vi "Destroy.vi"(8 "Error In":errorcluster, 11 "reference in":refnum<class "VdAnalogInput_Simulated.lvclass">) -> (0 "Error Out":errorcluster, 3 "reference out":refnum<class "VdAnalogInput_Simulated.lvclass">)   [LabVIEW 2020, in "VdAnalogInput_Simulated.lvclass"]
uses:
  VdAnalogInput_Simulated.lvclass
  VdAnalogInput_class/VdAnalogInput.lvclass
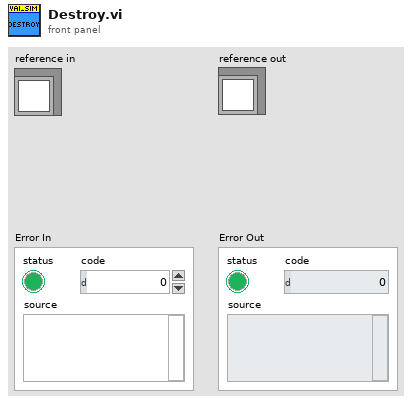
[diagram p1: front panel]
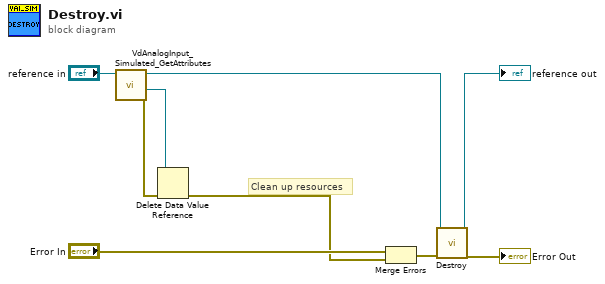
[diagram p0: block diagram]
diagram:
  # "Clean up resources"
  n1 = call "VdAnalogInput_Simulated_GetAttributes.vi"("reference in"="reference in") -> ("error out"=w7:errorcluster, "DataRef"=w5:refnum<data-value>, "reference out"=w6:refnum<class "VdAnalogInput_Simulated.lvclass">)  [unwired: 7 in, 1 out]
  n2 = Delete Data Value Reference(data value reference=w5, error in=w7) -> (error out=w1:errorcluster)  [unwired: 1 out]
  n3 = Merge Errors("Error In", w1) -> (w9:errorcluster)
  n4 = call-parent "Destroy.vi"("Error In"=w9, "reference in"=w6) -> ("Error Out"=→"Error Out":errorcluster, "reference out"=→"reference out":refnum<class "VdAnalogInput_Simulated.lvclass">)  [unwired: 8 in]
